vi "Smart Poultry Brooder System.vi"() -> ()   [LabVIEW 2022 SP3]
uses:
  <vilib>/DAQmx/read.llb/DAQmx Read (Analog 1D DBL NChan 1Samp).vi
  <vilib>/Analysis/baseanly.llb/Mean (DBL).vi
  <vilib>/DAQmx/read.llb/DAQmx Read (Analog DBL 1Chan 1Samp).vi
  <vilib>/DAQmx/create/channels.llb/DAQmx Create Channel (AI-Voltage-Basic).vi
  <vilib>/DAQmx/miscellaneous.llb/DAQmx Fill In Error Info.vi
  <vilib>/Utility/file.llb/Write Delimited Spreadsheet (string).vi
  <vilib>/Analysis/NI_AALBase.lvlib
panel:
  out "Thermometer":dbl(slide) scale=0.0..100.0
  out "End of Day":bool
  out "Weight Indicator":bool
  out "Initial Weight":dbl(knob) scale=0.0..1000.0
  out "Inside refilling loop":bool
  out "Still Level":dbl(slide) scale=0.0..8000.0
  out "filling voltage":dbl
  out "Filling Level":dbl(slide) scale=0.0..8000.0
  out "Voltage_L":dbl
  in  "Water level and weight":tag
  out "Voltage_W":dbl
  in  "SampleSize":u8=6
  out "Scale":dbl(knob) scale=0.0..1000.0
  out "Mean Voltage_W":dbl
  in  "Time Target (s)":dbl=20.0
  out "Time Taken (s)":dbl caption="Elapsed Time (s)"
  out "Status of the system":string
  out "Fan":bool
  in  "VISA resource name":refnum<visa-resource-name>
  out "Heating Element":bool
  out "Relative Humidity":dbl
  in  "Temp, humidity, weight":tag
  # "SMART POULTRY BROODER"
  # "Maintaining a controlled environment"
  # "Measuring Weight and Water Level"
  # "Refilling the tank"
  # "(60s)"
  # "Fixed Level = 4000ml"
  # "Weight value :"
  # "Fixed value = 600g"
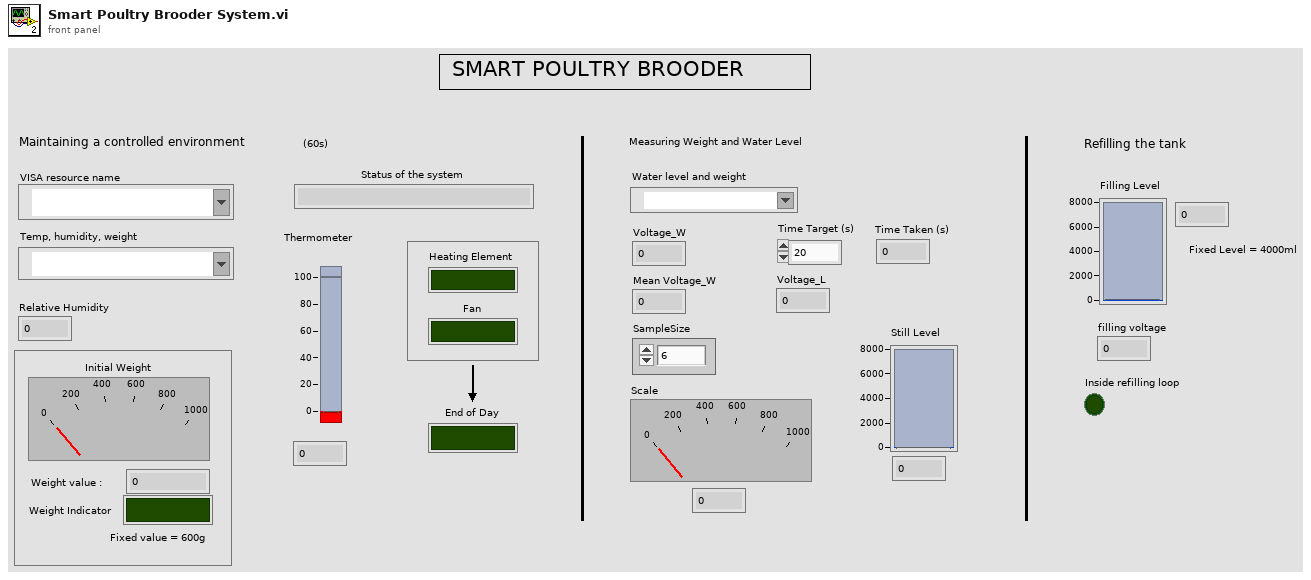
[diagram p1: front panel]
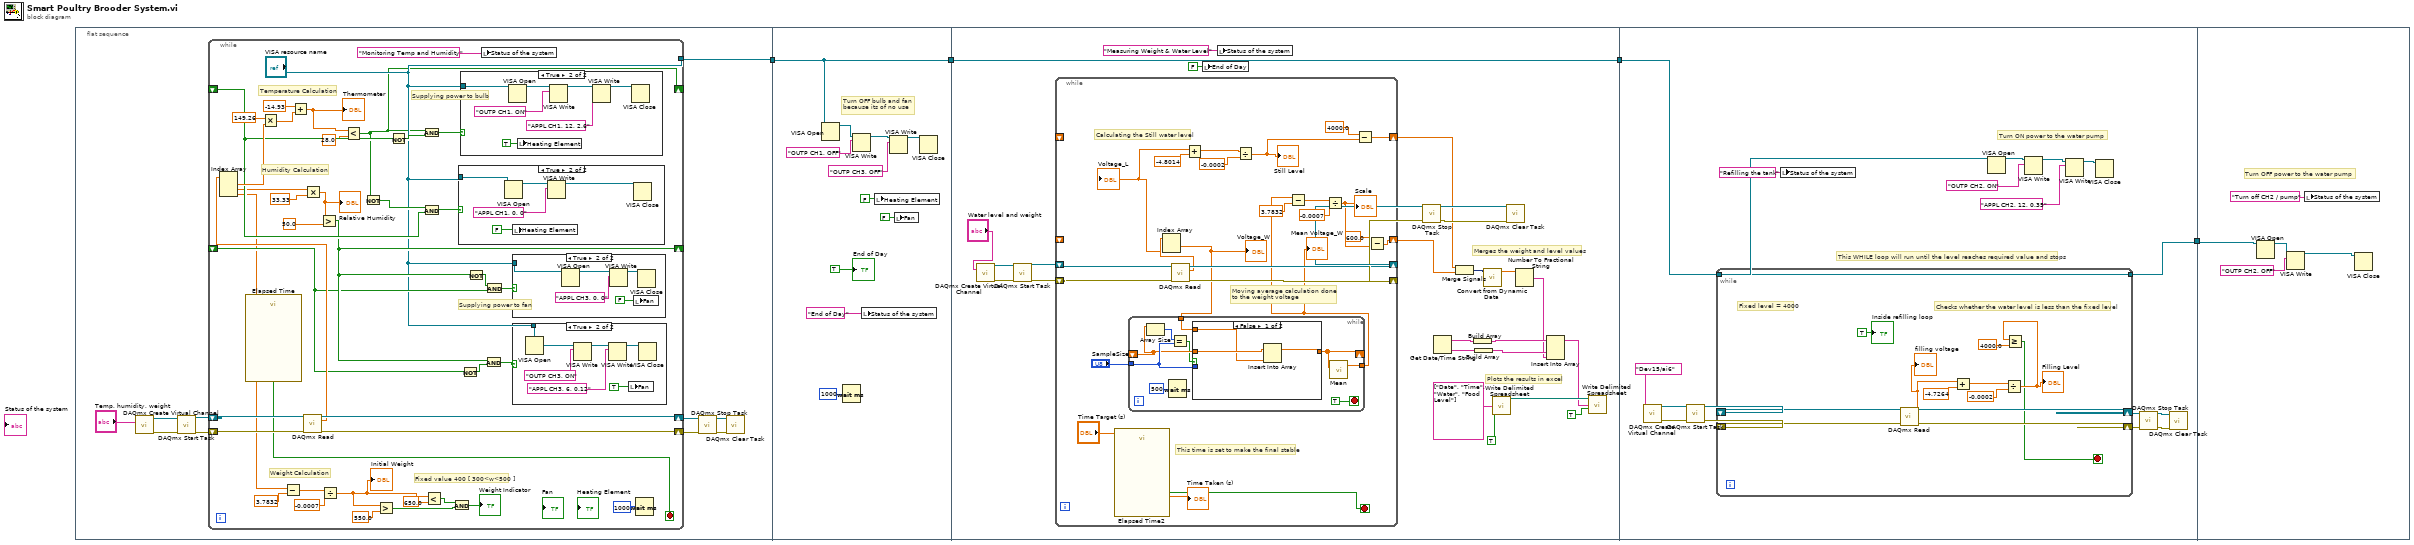
[diagram p0: block diagram]
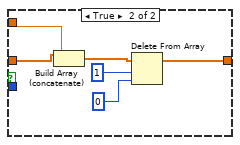
[diagram p6: hidden frame]
diagram:
  n1 = flat-sequence {
    tunnel: [w5] -> w4
    tunnel: w4 -> [w81]
    tunnel: [w81] -> w2
    tunnel: [w96] -> w3
    tunnel: w2 -> [w96]
    tunnel: w3 -> [w159]
    tunnel: [w165] -> w1
    tunnel: w1 -> [w192]
    frame #0 {
      n2 = call-poly <vilib>:"DAQmx Create Virtual Channel.vi"("physical channels"="Temp, humidity, weight") -> ("task out"=w14:refnum<k21>, "error out"=w10:errorcluster)  [unwired: 13 in]
      n3 = call <vilib>:"DAQmx Start Task.vi"("task/channels in"=w14, "error in"=w10) -> ("task out"=w13:refnum<k21>, "error out"=w9:errorcluster)  [unwired: 12 in]
      n4 = while {
        shift-right: [w53] -> w12
        shift-left: w13 -> [w55]
        shift-right: [w52] -> w8
        shift-left: w9 -> [w54]
        shift-right: [w15] -> _
        shift-left: _ -> [w44]
        shift-right: [w35] -> _
        shift-left: _ -> [w32]
        tunnel: ["VISA resource name"] -> w5
        stop <- w30 stop-if-true
        # "Weight Calculation"
        # "Supplying power to fan"
        # "Supplying power to bulb"
        # "Humidity Calculation"
        # "Temperature Calculation"
        # "Fixed value 400 [ 300<w<500 ]"
        n5 = call "Elapsed Time"() -> ("Time has Elapsed"=w30:bool)  [unwired: 12 in, 7 out]
        n6 = call-poly <vilib>:"DAQmx Read.vi"("task/channels in"=w55, "error in"=w54) -> ("task out"=w53:refnum<k21>, "data"=w51:dbl[], "error out"=w52:errorcluster)  [unwired: 11 in]
        n7 = Index Array(array=w51) -> (element #1=w50:dbl, element #2=w39:dbl, element #3=w24:dbl)  [unwired: 3 in]
        n8 = Multiply(x=149.26, y=w50) -> (x*y=w48:dbl)
        n9 = Subtract(x=w24, y=3.7832) -> (x-y=w27:dbl)
        n10 = Add(x=-14.93, y=w48) -> (x+y=w16:dbl)
        "Thermometer" <- w16
        n11 = Multiply(x=w39, y=33.33) -> (x*y=w38:dbl)
        "Relative Humidity" <- w38
        n12 = Greater?(x=w38, y=50.0) -> (0:w35:bool)
        n13 = Divide(x=w27, y=-0.0007) -> (x/y=w22:dbl)
        "Initial Weight" <- w22
        n14 = Less?(x=w16, y=28.0) -> (x < y?=w15:bool)
        n15 = Not(x=w15) -> (.not. x?=w43:bool)
        n16 = Greater?(x=w22, y=550.0) -> (0:w19:bool)
        n17 = Not(x=w44) -> (.not. x?=w45:bool)
        n18 = And(x=w15, y=w45) -> (x .and. y?=w46:bool)
        n19 = And(x=w43, y=w44) -> (x .and. y?=w42:bool)
        n20 = Less?(x=w22, y=650.0) -> (x < y?=w20:bool)
        n21 = And(x=w20, y=w19) -> (x .and. y?=→"Weight Indicator":bool)
        n22 = case shown="True" w42 {
          tunnel: "VISA resource name" -> [_ w68]
          frame False {
          }
          frame True {
            n23 = VISA Open(VISA resource name=w68) -> (VISA resource name=w72:refnum<visa-resource-name>)  [unwired: 4 in, 1 out]
            n24 = local write "Heating Element"(FALSE) -> ()
            n25 = VISA Write(VISA resource name=w72, write buffer="APPL CH1, 0, 0") -> (VISA resource name out=w69:refnum<visa-resource-name>)  [unwired: 1 in, 2 out]
            n26 = VISA Close(VISA resource name=w69) -> ()  [unwired: 1 in, 1 out]
          }
        }
        n27 = case shown="True" w46 {
          tunnel: "VISA resource name" -> [_ w73]
          frame False {
          }
          frame True {
            n28 = VISA Open(VISA resource name=w73) -> (VISA resource name=w78:refnum<visa-resource-name>)  [unwired: 4 in, 1 out]
            n29 = local write "Heating Element"(TRUE) -> ()
            n30 = VISA Write(VISA resource name=w78, write buffer="OUTP CH1, ON") -> (VISA resource name out=w76:refnum<visa-resource-name>)  [unwired: 1 in, 2 out]
            n31 = VISA Write(VISA resource name=w76, write buffer="APPL CH1, 12, 2.6") -> (VISA resource name out=w74:refnum<visa-resource-name>)  [unwired: 1 in, 2 out]
            n32 = VISA Close(VISA resource name=w74) -> ()  [unwired: 1 in, 1 out]
          }
        }
        n33 = Not(x=w32) -> (.not. x?=w36:bool)
        n34 = Not(x=w35) -> (.not. x?=w33:bool)
        n35 = local write "Status of the system"("Monitoring Temp and Humidity") -> ()
        n36 = And(x=w35, y=w36) -> (x .and. y?=w31:bool)
        n37 = And(x=w33, y=w32) -> (x .and. y?=w34:bool)
        n38 = case shown="True" w34 {
          tunnel: "VISA resource name" -> [_ w57]
          frame False {
          }
          frame True {
            n39 = VISA Open(VISA resource name=w57) -> (VISA resource name=w60:refnum<visa-resource-name>)  [unwired: 4 in, 1 out]
            n40 = VISA Write(VISA resource name=w60, write buffer="APPL CH3, 0, 0") -> (VISA resource name out=w59:refnum<visa-resource-name>)  [unwired: 1 in, 2 out]
            n41 = local write "Fan"(FALSE) -> ()
            n42 = VISA Close(VISA resource name=w59) -> ()  [unwired: 1 in, 1 out]
          }
        }
        n43 = case shown="True" w31 {
          tunnel: "VISA resource name" -> [_ w67]
          frame False {
          }
          frame True {
            n44 = VISA Open(VISA resource name=w67) -> (VISA resource name=w66:refnum<visa-resource-name>)  [unwired: 4 in, 1 out]
            n45 = VISA Write(VISA resource name=w66, write buffer="OUTP CH3, ON") -> (VISA resource name out=w65:refnum<visa-resource-name>)  [unwired: 1 in, 2 out]
            n46 = VISA Write(VISA resource name=w65, write buffer="APPL CH3, 6, 0.12") -> (VISA resource name out=w62:refnum<visa-resource-name>)  [unwired: 1 in, 2 out]
            n47 = local write "Fan"(TRUE) -> ()
            n48 = VISA Close(VISA resource name=w62) -> ()  [unwired: 1 in, 1 out]
          }
        }
        n49 = Wait (ms)(milliseconds to wait=u32 1000) -> ()  [unwired: 1 out]
      }
      n50 = call <vilib>:"DAQmx Stop Task.vi"("task/channels in"=w12, "error in"=w8) -> ("task out"=w11:refnum<k21>, "error out"=w7:errorcluster)  [unwired: 12 in]
      n51 = call <vilib>:"DAQmx Clear Task.vi"("task in"=w11, "error in"=w7) -> ()  [unwired: 13 in, 1 out]
    }
    frame #1 {
      # "Turn OFF bulb and fan \nbecause its of no use"
      n52 = VISA Open(VISA resource name=w81) -> (VISA resource name=w90:refnum<visa-resource-name>)  [unwired: 4 in, 1 out]
      n53 = Wait (ms)(milliseconds to wait=u32 1000) -> ()  [unwired: 1 out]
      n54 = VISA Write(VISA resource name=w90, write buffer="OUTP CH1, OFF") -> (VISA resource name out=w87:refnum<visa-resource-name>)  [unwired: 1 in, 2 out]
      n55 = local write "Status of the system"("End of Day") -> ()
      n56 = local write "Heating Element"(FALSE ("Heating Element")) -> ()
      n57 = VISA Write(VISA resource name=w87, write buffer="OUTP CH3, OFF") -> (VISA resource name out=w86:refnum<visa-resource-name>)  [unwired: 1 in, 2 out]
      n58 = local write "Fan"(FALSE ("Fan")) -> ()
      n59 = VISA Close(VISA resource name=w86) -> ()  [unwired: 1 in, 1 out]
      "End of Day" <- TRUE ("End of Day")
    }
    frame #2 {
      # "Plots the results in excel"
      # "Merges the weight and level values"
      n60 = call-poly <vilib>:"DAQmx Create Virtual Channel.vi"("physical channels"="Water level and weight") -> ("task out"=w114:refnum<k21>, "error out"=w110:errorcluster)  [unwired: 13 in]
      n61 = call <vilib>:"DAQmx Start Task.vi"("task/channels in"=w114, "error in"=w110) -> ("task out"=w113:refnum<k21>, "error out"=w109:errorcluster)  [unwired: 12 in]
      n62 = while {
        shift-right: [w137] -> w112
        shift-left: w113 -> [w140]
        shift-right: [w138] -> w108
        shift-left: w109 -> [w139]
        shift-right: [w118] -> w94
        shift-left: _ -> [_]
        shift-right: [w122] -> w93
        shift-left: _ -> [_]
        stop <- w133 stop-if-true
        # "This time is set to make the final stable"
        # "Moving average calculation done \nto the weight voltage"
        # "Calculating the Still water level"
        n63 = call "Elapsed Time2"("Time Target (s)"="Time Target (s)") -> ("Elapsed Time (s)"=→"Time Taken (s)":dbl, "Time has Elapsed"=w133:bool)  [unwired: 11 in, 6 out]
        n64 = call-poly <vilib>:"DAQmx Read.vi"("task/channels in"=w140, "error in"=w139) -> ("task out"=w137:refnum<k21>, "data"=w128:dbl[], "error out"=w138:errorcluster)  [unwired: 11 in]
        n65 = Index Array(array=w128) -> (element #1=w127:dbl, element #2=w123:dbl)  [unwired: 2 in]
        "Voltage_W" <- w127
        "Voltage_L" <- w123
        n66 = while {
          tunnel: w127 -> [w149]
          tunnel: "SampleSize" -> [w147]
          shift-right: [w143] -> _
          shift-left: _ -> [w146]
          tunnel: [w142] -> w129
          stop <- TRUE stop-if-true
          n67 = Array Size(array=w146) -> (size(s)=w148:i32)
          n68 = Wait (ms)(milliseconds to wait=u32 500) -> ()  [unwired: 1 out]
          n69 = Equal?(x=w148, y=w147) -> (x = y?=w141:bool)
          n70 = case shown="False" w141 {
            tunnel: w149 -> [w150 w158]
            tunnel: [w152 w156] -> w143
            tunnel: w146 -> [w151 w155]
            tunnel: w147 -> [_ _]
            frame False {
              n71 = Insert Into Array(array=w151, new element=w150) -> (w152:dbl[])  [unwired: 1 in]
            }
            frame True {
              n72 = Build Array (concatenate)(w155, w158) -> (w157:dbl[])
              n73 = Delete From Array(array=w157, length=1, index=0) -> (array with subset deleted=w156:dbl[])  [unwired: 1 out]
            }
          }
          n74 = call-poly <vilib>:"Mean.vi"("X"=w143) -> ("mean"=w142:dbl)  [unwired: 1 out]
        }
        "Mean Voltage_W" <- w129
        n75 = Add(x=w123, y=-4.8014) -> (x+y=w125:dbl)
        n76 = Divide(x=w125, y=-0.0002) -> (x/y=w121:dbl)
        "Still Level" <- w121
        n77 = Subtract(x=w129, y=3.7832) -> (x-y=w136:dbl)
        n78 = Divide(x=w136, y=-0.0007) -> (x/y=w119:dbl)
        "Scale" <- w119
        n79 = Subtract(x=4000.0, y=w121) -> (x-y=w122:dbl)
        n80 = Subtract(x=600.0, y=w119) -> (x-y=w118:dbl)
      }
      n81 = local write "End of Day"(FALSE ("End of Day")) -> ()
      n82 = local write "Status of the system"("Measuring Weight & Water Level" ("Status of the system")) -> ()
      n83 = call <vilib>:"DAQmx Stop Task.vi"("task/channels in"=w112, "error in"=w108) -> ("task out"=w111:refnum<k21>, "error out"=w107:errorcluster)  [unwired: 12 in]
      n84 = Get Date/Time String() -> (date string=w106:string, time string=w105:string)  [unwired: 3 in]
      n85 = Merge Signals(w93, w94) -> (w92:dynamicdata)
      n86 = Build Array(w106) -> (w104:string[])
      n87 = Build Array(w105) -> (w103:string[])
      n88 = call "Convert from Dynamic Data"("Dynamic Data Type"=w92) -> ("Array"=w91:dbl[])  [unwired: 3 in]
      n89 = call-poly <vilib>:"Write Delimited Spreadsheet.vi"("1D data"=string[] ["Date", "Time", "Water", "Food Level"], "append to file? (new file:F)"=TRUE) -> ("new file path (Not A Path if cancelled)"=w101:path)  [unwired: 12 in, 1 out]
      n90 = call <vilib>:"DAQmx Clear Task.vi"("task in"=w111, "error in"=w107) -> ()  [unwired: 13 in, 1 out]
      n91 = Number To Fractional String(number=w91) -> (F-format string=w99:string[])  [unwired: 3 in]
      n92 = Insert Into Array(array=w104, new element #1=w103, new element #2=w99) -> (w100:string[])  [unwired: 1 in]
      n93 = call-poly <vilib>:"Write Delimited Spreadsheet.vi"("file path (dialog if empty)"=w101, "1D data"=w100, "append to file? (new file:F)"=TRUE) -> ()  [unwired: 11 in, 2 out]
    }
    frame #3 {
      # "This WHILE loop will run until the level reaches required value and stops"
      # "Turn ON power to the water pump"
      n94 = call-poly <vilib>:"DAQmx Create Virtual Channel.vi"("physical channels"=tag "Dev15/ai6") -> ("task out"=w174:refnum<k21>, "error out"=w170:errorcluster)  [unwired: 13 in]
      n95 = call <vilib>:"DAQmx Start Task.vi"("task/channels in"=w174, "error in"=w170) -> ("task out"=w173:refnum<k21>, "error out"=w169:errorcluster)  [unwired: 12 in]
      n96 = while {
        shift-right: [w186] -> w172
        shift-left: w173 -> [w188]
        shift-right: [w185] -> w168
        shift-left: w169 -> [w187]
        tunnel: w159 -> [w184]
        tunnel: [w184] -> w165
        stop <- w177 stop-if-true
        # "Checks whether the water level is less than the fixed level"
        # "Fixed level = 4000"
        n97 = call-poly <vilib>:"DAQmx Read.vi"("task/channels in"=w188, "error in"=w187) -> ("task out"=w186:refnum<k21>, "data"=w180:dbl, "error out"=w185:errorcluster)  [unwired: 11 in]
        "filling voltage" <- w180
        n98 = Add(x=w180, y=-4.7264) -> (x+y=w182:dbl)
        n99 = Divide(x=w182, y=-0.0002) -> (x/y=w179:dbl)
        "Filling Level" <- w179
        n100 = Greater Or Equal?(x=w179, y=4000.0) -> (x >= y?=w177:bool)
        "Inside refilling loop" <- TRUE ("Inside refilling loop")
      }
      n101 = local write "Status of the system"("Refilling the tank" ("Status of the system")) -> ()
      n102 = VISA Open(VISA resource name=w159) -> (VISA resource name=w162:refnum<visa-resource-name>)  [unwired: 4 in, 1 out]
      n103 = VISA Write(VISA resource name=w162, write buffer="OUTP CH2, ON") -> (VISA resource name out=w163:refnum<visa-resource-name>)  [unwired: 1 in, 2 out]
      n104 = VISA Write(VISA resource name=w163, write buffer="APPL CH2, 12, 0.35") -> (VISA resource name out=w164:refnum<visa-resource-name>)  [unwired: 1 in, 2 out]
      n105 = VISA Close(VISA resource name=w164) -> ()  [unwired: 1 in, 1 out]
      n106 = call <vilib>:"DAQmx Stop Task.vi"("task/channels in"=w172, "error in"=w168) -> ("task out"=w171:refnum<k21>, "error out"=w167:errorcluster)  [unwired: 12 in]
      n107 = call <vilib>:"DAQmx Clear Task.vi"("task in"=w171, "error in"=w167) -> ()  [unwired: 13 in, 1 out]
    }
    frame #4 {
      # "Turn OFF power to the water pump"
      n108 = VISA Open(VISA resource name=w192) -> (VISA resource name=w191:refnum<visa-resource-name>)  [unwired: 4 in, 1 out]
      n109 = VISA Write(VISA resource name=w191, write buffer="OUTP CH2, OFF") -> (VISA resource name out=w190:refnum<visa-resource-name>)  [unwired: 1 in, 2 out]
      n110 = local write "Status of the system"("Turn off CH2 / pump" ("Status of the system")) -> ()
      n111 = VISA Close(VISA resource name=w190) -> ()  [unwired: 1 in, 1 out]
    }
  }
